vi "VRM Cartesian to Spherical.vi"(8 "error in (no error)":errorcluster, 11 "Field (x,y,z)":dbl[](array[numeric])) -> (0 "error out":errorcluster, 3 "Field (r,theta,phi)":dbl[](array[numeric]))   [LabVIEW 2019, in "Instrument.OxfordVRM.lvclass"]
uses:
  Instrument.OxfordVRM.lvclass
  <vilib>/Analysis/coordinate.llb/3D Coordinate Conversion (Scalar).vi
  <vilib>/Analysis/NI_AALPro.lvlib
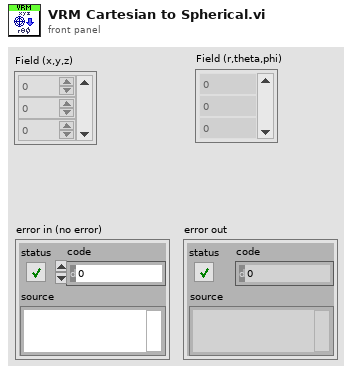
[diagram p1: front panel]
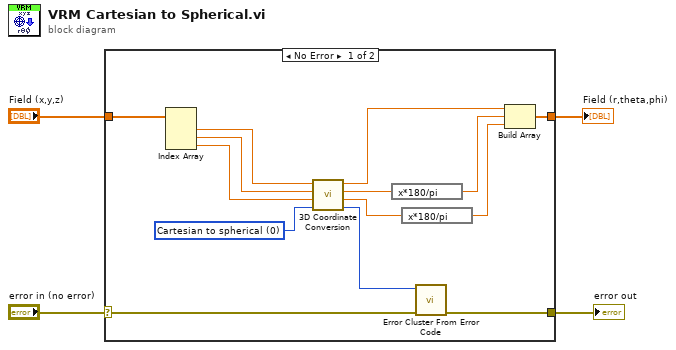
[diagram p0: block diagram]
diagram:
  n1 = case shown="No Error" "error in (no error)" {
    selector: "error in (no error)" -> [w14 w19]
    tunnel: [w13 w19] -> w3
    tunnel: "Field (x,y,z)" -> [w12 _]
    tunnel: [w5 _] -> w1
    frame No Error {
      w18 = u16 0 items=["Cartesian to spherical", "spherical to Cartesian", "Cartesian to cylindrical", "cylindrical to Cartesian", "spherical to cylindrical", "cylindrical to spherical"] ("conversion type")
      n2 = Index Array(array=w12) -> (element #1=w11:dbl, element #2=w10:dbl, element #3=w9:dbl)  [unwired: 3 in]
      n3 = call-poly <vilib>:"3D Coordinate Conversion.vi"("conversion type"=w18, "axis 3"=w9, "axis 2"=w10, "axis 1"=w11) -> ("error"=w15:i32, "axis 3 out"=w17:dbl, "axis 2 out"=w16:dbl, "axis 1 out"=w8:dbl)  [unwired: 4 in]
      n4 = expression code="x*180/pi"(w16) -> (w7:dbl)
      n5 = expression code="x*180/pi"(w17) -> (w6:dbl)
      n6 = call <vilib>:"Error Cluster From Error Code.vi"("error in (no error)"=w14, "error code (0)"=w15) -> ("error out"=w13:errorcluster)  [unwired: 7 in]
      n7 = Build Array(w8, w7, w6) -> (w5:dbl[])
    }
    frame Error {
    }
  }
  "error out" <- w3
  "Field (r,theta,phi)" <- w1
